vi "addNode.vi"(0 "reference":refnum<class "AbstractNode.lvclass">, 1 "node":refnum<class "AbstractNode.lvclass">, 2 "point2D":T1 {"y" format="%.2f"; "x" format="%.2f"}, 5 "error in (no error)":errorcluster) -> (14 "reference out":refnum<class "AbstractNode.lvclass">, 15 "added":bool, 19 "error out":errorcluster)   [LabVIEW 2012, in "AbstractNode.lvclass"]
doc: "public boolean addNode(Node n, Point2D p)"
uses:
  <resource>/Framework/Providers/Open_GDS/UML/AbstractNode_class/AbstractNode.lvclass
  <resource>/Framework/Providers/Open_GDS/UML/General/Point/Point Point2D.ctl
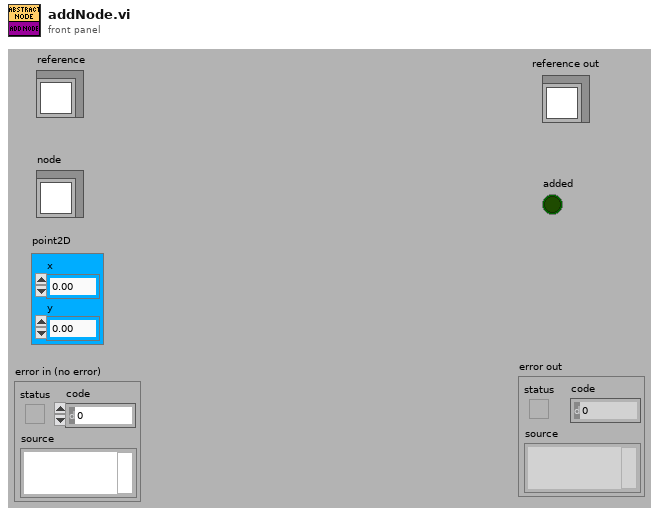
[diagram p1: front panel]
types:
  T1 = typedef "Point Point2D.ctl" = cluster{"x":dbl, "y":dbl}
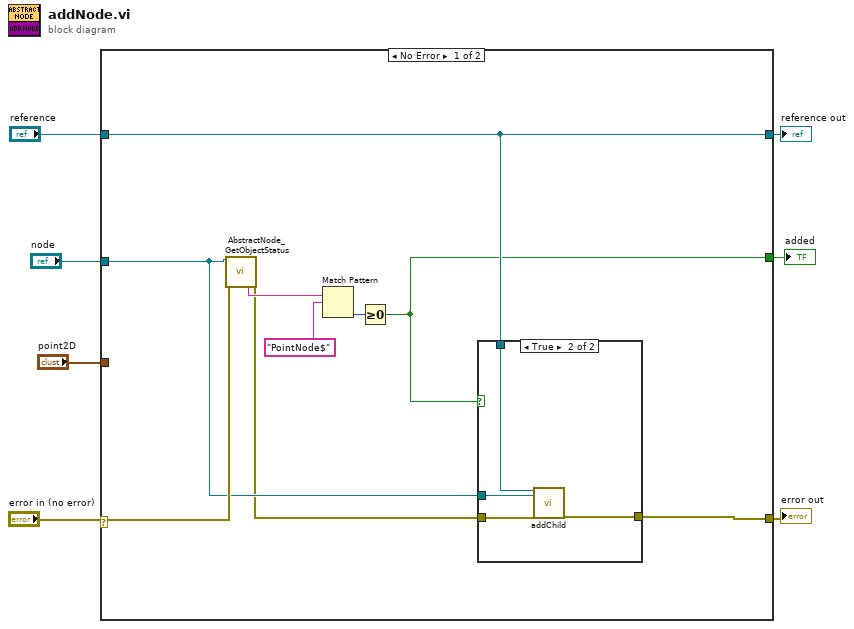
[diagram p0: block diagram]
diagram:
  n1 = case shown="No Error" "error in (no error)" {
    selector: "error in (no error)" -> [w14 w22]
    tunnel: "reference" -> [w16 w23]
    tunnel: [w15 w22] -> w6
    tunnel: [w16 w23] -> w5
    tunnel: "node" -> [w13 _]
    tunnel: "point2D" -> [_ _]
    tunnel: [w12 _] -> w1
    frame No Error {
      n2 = call <resource>:"AbstractNode_GetObjectStatus.vi"("reference in"=w13, "error in (no error)"=w14) -> ("Class name"=w11:string, "error out"=w9:errorcluster)  [unwired: 16 out]
      n3 = Match Pattern(string=w11, regular expression="PointNode$" ("y")) -> (offset past match=w8:i32)  [unwired: 4 out]
      n4 = Greater Or Equal To 0?(x=w8) -> (x >= 0?=w12:bool)
      n5 = case shown="True" w12 {
        tunnel: w9 -> [w17 w21]
        tunnel: [w17 w20] -> w15
        tunnel: w16 -> [_ w19]
        tunnel: w13 -> [_ w18]
        frame False {
        }
        frame True {
          n6 = call-dynamic "addChild.vi"("reference"=w19, "node"=w18, "error in (no error)"=w21) -> ("error out"=w20:errorcluster)  [unwired: 15 in, 1 out]
        }
      }
    }
    frame Error {
    }
  }
  "reference out" <- w5
  "error out" <- w6
  "added" <- w1
